vi "MaketabTest.vi"(9 "nbmodule":i32=8, 10 "TCell":string, 11 "VCell":string) -> (1 "nbCMU":i8, 2 "Tcell":dbl[][](array[numeric]), 3 "Vcell":dbl[][](array[numeric]))   [LabVIEW 2020]
panel:
  # ":6.1ms \n\n IC 1: GPIO-1:1.2477, GPIO-2:1.7051, GPIO-3:1.2580, GPIO-4:1.7074, GPIO-5:2.9079, Vref2:3.0032\n IC 2: GPIO-1:1.2521, GPIO-2:1.7085, GPIO-3:1.2560, GPIO-4:1.7032, GPIO-5:2.9121, Vref2:3.0050\n IC 3: GPIO-1:1.2455, GPIO-2:1.7066, GPIO-3:1.2587, GPIO-4:1.7098, GPIO-5:2.9086, Vref2:3.0028\n IC 4: GPIO-1:1.2512, GPIO-2:1.7130, GPIO-3:1.2503, GPIO-4:1.6984, GPIO-5:2.9110, Vref2:3.0040\n IC 5: GPIO-1:1.2579, GPIO-2:1.7092, GPIO-3:1.2628, GPIO-4:1.7040, GPIO-5:2.9101, Vref2:3.0045\n IC 6: GPIO-1:1.2485, GPIO-2:1.7137, GPIO-3:1.2526, GPIO-4:1.7087, GPIO-5:2.9080, Vref2:3.0032\n IC 7: GPIO-1:1.2482, GPIO-2:1.7069, GPIO-3:1.2553, GPIO-4:1.7074, GPIO-5:2.9110, Vref2:3.0053\n IC 8: GPIO-1:1.2587, GPIO-2:1.7070, GPIO-3:1.2489, GPIO-4:1.7048, GPIO-5:2.9078, Vref2:3.0028\n IC 9: GPIO-1:1.2436, GPIO-2:1.7067, GPIO-3:1.2504, GPIO-4:1.6995, GPIO-5:2.9091, Vref2:3.0050\n IC 10: GPIO-1:1.2518, GPIO-2:1.6997, GPIO-3:1.2551, GPIO-4:1.7011, GPIO-5:2.9095, Vref2:3.0048\n IC 11: GPIO-1:1.2488, GPIO-2:1.7019, GPIO-3:1.2500, GPIO-4:1.7059, GPIO-5:2.9073, Vref2:3.0024\n IC 12: GPIO-1:1.2540, GPIO-2:1.7065, GPIO-3:1.2515, GPIO-4:1.7009, GPIO-5:2.9122, Vref2:3.0053\n IC 13: GPIO-1:1.2449, GPIO-2:1.6945, GPIO-3:1.2550, GPIO-4:1.7049, GPIO-5:2.9070, Vref2:3.0026\n IC 14: GPIO-1:1.2529, GPIO-2:1.6994, GPIO-3:1.2502, GPIO-4:1.7044, GPIO-5:2.9082, Vref2:3.0037\n IC 15: GPIO-1:1.2406, GPIO-2:1.7071, GPIO-3:3.0023, GPIO-4:3.0029, GPIO-5:2.9109, Vref2:3.0045\n IC 16: GPIO-1:6.5535, GPIO-2:6.5535, GPIO-3:6.5535, GPIO-4:6.5535, GPIO-5:6.5535, Vref2:6.5535\n\n\n IC 1:  C1:3.5980, C2:3.5975, C3:3.5982, C4:3.5996, C5:3.5962, C6:3.5999, C7:3.5986, C8:3.6013, C9:3.5949, C10:3.5974, C11:3.5987, C12:3.5993,\n IC 2:  C1:3.5974, C2:3.5966, C3:3.5979, C4:3.5976, C5:3.5964, C6:3.5976, C7:3.5942, C8:3.5990, C9:3.5944, C10:3.5943, C11:3.5963, C12:3.5960,\n IC 3:  C1:3.6022, C2:3.5980, C3:3.5952, C4:3.5972, C5:3.5980, C6:3.5971, C7:3.5959, C8:3.5939, C9:3.5937, C10:3.5963, C11:3.5922, C12:3.5966,\n IC 4:  C1:3.5975, C2:3.5963, C3:3.5980, C4:3.5990, C5:3.5991, C6:3.5976, C7:3.5952, C8:3.5965, C9:3.5960, C10:3.5962, C11:3.5925, C12:3.5965,\n IC 5:  C1:3.5963, C2:3.5979, C3:3.5985, C4:3.5950, C5:3.5964, C6:3.5994, C7:3.5961, C8:3.6015, C9:3.5992, C10:3.5991, C11:3.5964, C12:3.5992,\n IC 6:  C1:3.6011, C2:3.5998, C3:3.5995, C4:3.5991, C5:3.5997, C6:3.6012, C7:3.6004, C8:3.6028, C9:3.5988, C10:3.5994, C11:3.5980, C12:3.6006,\n IC 7:  C1:3.6003, C2:3.6004, C3:3.5966, C4:3.6022, C5:3.5981, C6:3.6015, C7:3.5966, C8:3.5980, C9:3.5971, C10:3.5974, C11:3.5963, C12:3.5975,\n IC 8:  C1:3.5990, C2:3.6002, C3:3.6004, C4:3.6009, C5:3.5985, C6:3.6008, C7:3.5981, C8:3.5980, C9:3.5962, C10:3.6008, C11:3.5968, C12:3.5974,\n IC 9:  C1:3.6010, C2:3.5984, C3:3.5993, C4:3.5979, C5:3.6001, C6:3.5976, C7:3.6003, C8:3.5980, C9:3.5973, C10:3.5967, C11:3.5981, C12:3.5999,\n IC 10:  C1:3.5960, C2:3.5992, C3:3.5991, C4:3.5977, C5:3.5976, C6:3.5970, C7:3.5993, C8:3.6007, C9:3.5986, C10:3.6011, C11:3.6001, C12:3.6011,\n IC 11:  C1:3.5989, C2:3.5954, C3:3.5985, C4:3.5964, C5:3.5974, C6:3.5959, C7:3.5992, C8:3.5999, C9:3.5988, C10:3.5981, C11:3.5998, C12:3.5950,\n IC 12:  C1:3.5966, C2:3.5964, C3:3.5974, C4:3.5977, C5:3.5979, C6:3.6003, C7:3.5928, C8:3.5969, C9:3.5976, C10:3.5919, C11:3.5973, C12:3.5967,\n IC 13:  C1:3.5984, C2:3.5961, C3:3.5976, C4:3.5969, C5:3.5955, C6:3.5987, C7:3.5995, C8:3.5982, C9:3.5954, C10:3.5976, C11:3.5987, C12:3.5969,\n IC 14:  C1:3.5982, C2:3.5949, C3:3.5973, C4:3.5976, C5:3.5975, C6:3.5982, C7:3.6014, C8:3.5984, C9:3.5990, C10:3.5966, C11:3.5996, C12:3.5982,\n IC 15:  C1:3.6003, C2:3.5964, C3:3.5966, C4:0.0000, C5:0.0000, C6:0.0000, C7:3.5982, C8:3.5993, C9:3.5979, C10:0.0001, C11:0.0000, C12:0.0000,\n IC 16:  C1:6.5535, C2:6.5535, C3:6.5535, C4:6.5535, C5:6.5535, C6:6.5535, C7:6.5535, C8:6.5535, C9:6.5535, C10:6.5535, C11:6.5535, C12:6.5535,"
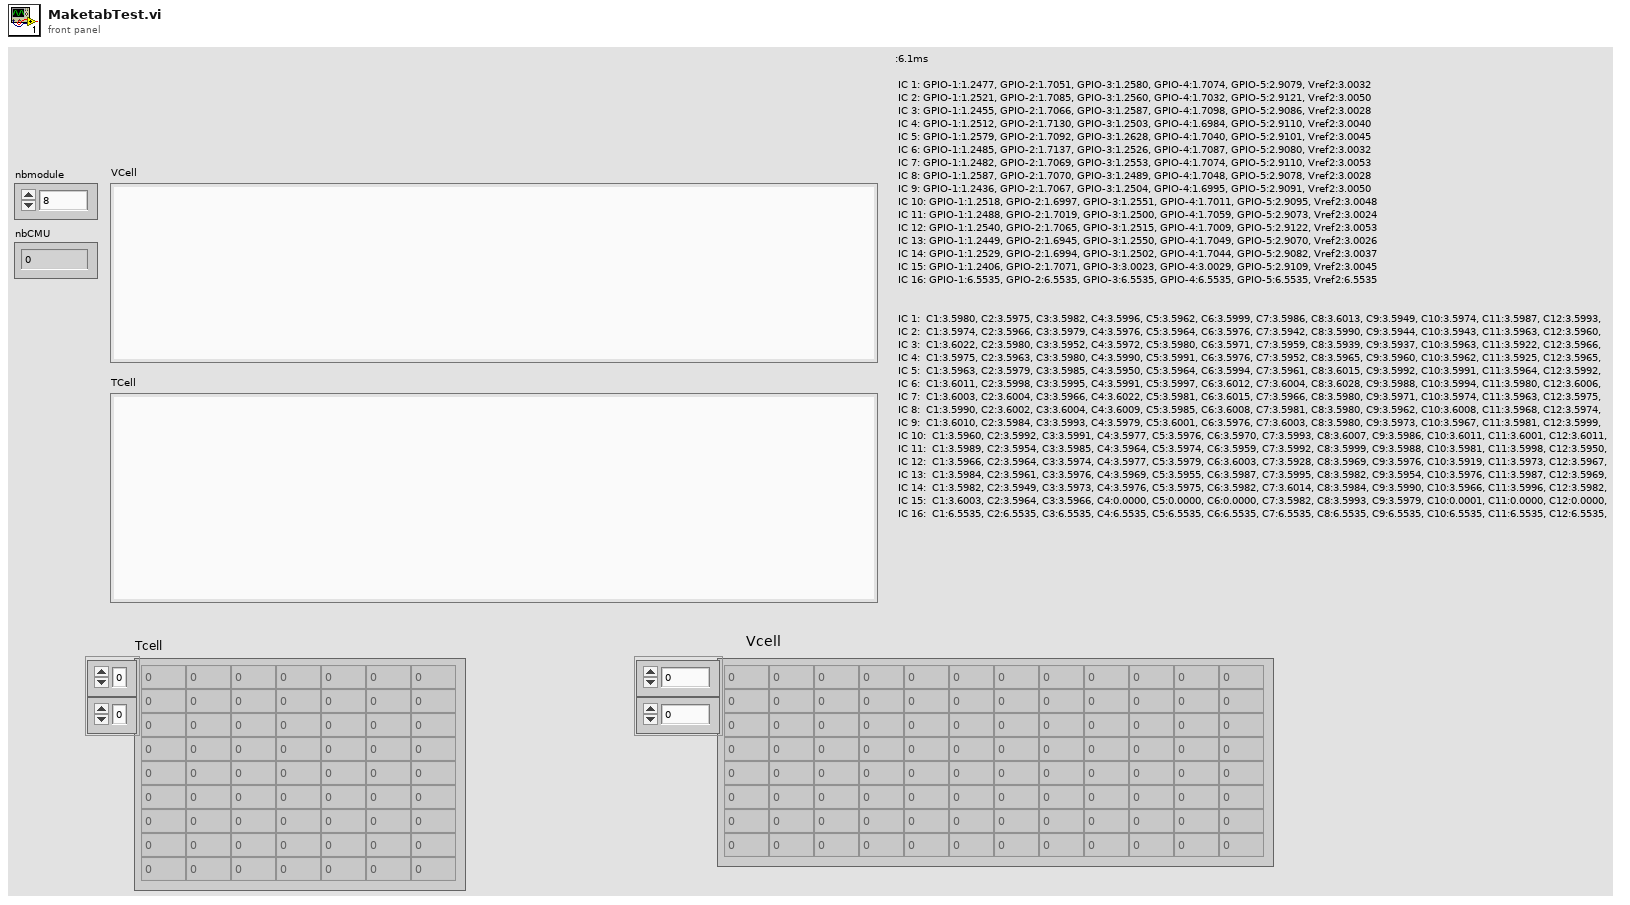
[diagram p1: front panel]
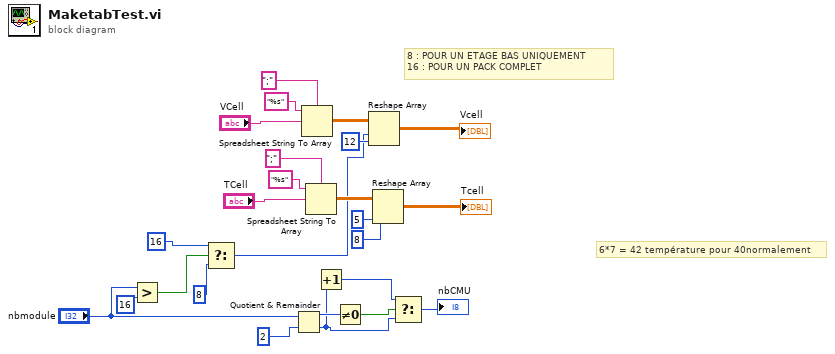
[diagram p0: block diagram]
diagram:
  # "6*7 = 42 température pour 40normalement"
  # "8 : POUR UN ETAGE BAS UNIQUEMENT\n16 : POUR UN PACK COMPLET"
  n1 = Greater?(x="nbmodule", y=16) -> (0:w4:bool)
  n2 = Select(t=16 ("y"), s=w4, f=8) -> (s? t:f=w1:i32)
  n3 = Quotient & Remainder(x="nbmodule", y=2) -> (x-y*floor(x/y)=w22:i32, floor(x/y)=w14:i32)
  n4 = Spreadsheet String To Array ("Chaîne au format tableur en tableau")(delimiter (Tab)=";" ("séparateur (Tabulation)"), format string="%s" ("chaîne de format"), spreadsheet string="VCell") -> (array=w17:dbl[][])  [unwired: 1 in]
  n5 = Spreadsheet String To Array ("Chaîne au format tableur en tableau")(delimiter (Tab)=";" ("séparateur (Tabulation)"), format string="%s" ("chaîne de format"), spreadsheet string="TCell") -> (array=w11:dbl[][])  [unwired: 1 in]
  n6 = Increment(x=w14) -> (x+1=w20:i32)
  n7 = Not Equal To 0?(x=w22) -> (x != 0?=w21:bool)
  n8 = Reshape Array(w17, w1, 12 ("taille de la dimension")) -> (→"Vcell":dbl[][])
  n9 = Reshape Array(w11, 8 ("taille de la dimension"), 5 ("taille de la dimension")) -> (→"Tcell":dbl[][])
  n10 = Select(t=w20, s=w21, f=w14) -> (s? t:f=→"nbCMU":i32)
